vi "Toggle Controls.vi"(2 "Exclude Controls":string[](array[string])=["Drive Live Controls Move Start"], 3 "Karteikartenreiter Referenz":refnum<vi>) -> ()   [LabVIEW 2010]
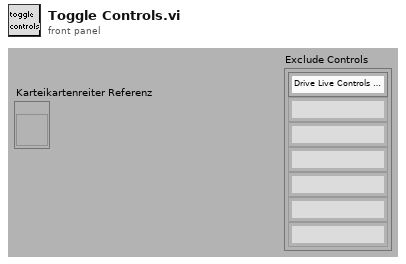
[diagram p1: front panel]
types:
  T1 = enum8{"Enabled", "Disabled", "Disabled and Grayed Out"}
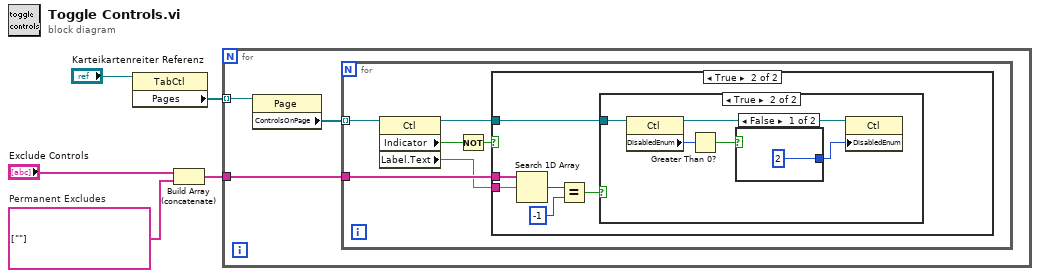
[diagram p0: block diagram]
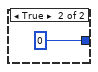
[diagram p4: hidden frame]
diagram:
  w5 = string[] [""]  # Permanent Excludes
  n1 = property class="TabCtl"(reference="Karteikartenreiter Referenz") -> ("Pages"=w4:refnum<vi>[])  [unwired: 1 in, 2 out]
  n2 = Build Array (concatenate)("Exclude Controls", w5) -> (w3:string[])
  n3 = for {
    tunnel: w4 -> [w8] mode=indexing
    tunnel: w3 -> [w6]
    n4 = property class="Page"(reference=w8) -> ("ControlsOnPage"=w7:refnum<vi>[])  [unwired: 1 in, 2 out]
    n5 = for {
      tunnel: w7 -> [w14] mode=indexing
      tunnel: w6 -> [w13]
      n6 = property class="Ctl"(reference=w14) -> (reference out=w12:refnum<vi>, "Indicator"=w9:bool, "Label.Text"=w10:string)  [unwired: 1 in, 1 out]
      n7 = Not(x=w9) -> (.not. x?=w11:bool)
      n8 = case shown="True" w11 {
        tunnel: w13 -> [_ w18]
        tunnel: w12 -> [_ w17]
        tunnel: w10 -> [_ w16]
        frame False {
        }
        frame True {
          n9 = Search 1D Array(1D array=w18, element=w16) -> (index of element=w19:i32)  [unwired: 1 in]
          n10 = Equal?(x=w19, y=-1) -> (x = y?=w15:bool)
          n11 = case shown="True" w15 {
            tunnel: w17 -> [_ w25]
            frame False {
            }
            frame True {
              n12 = property class="Ctl"(reference=w25) -> (reference out=w22:refnum<vi>, "DisabledEnum"=w24:T1)  [unwired: 1 in, 1 out]
              n13 = Greater Than 0?(x=w24) -> (x > 0?=w23:bool)
              n14 = case shown="False" w23 {
                tunnel: [2 ("y") 0 ("y")] -> w21
                frame False {
                }
                frame True {
                }
              }
              n15 = property class="Ctl"(reference=w22, "DisabledEnum"=w21) -> ()  [unwired: 1 in, 2 out]
            }
          }
        }
      }
    }
  }
